vi "Identificação MIMO.vi"(6 "System Order":i32=4, 7 "Remove Trend":bool, 8 "Init Pump 2 voltage":dbl=3.0 min=0.0 format="%.2f", 9 "Init Pump 1 voltage":dbl=3.0 min=0.0 format="%.2f", 11 "Stimulus and Response Signal":dbl[][](array[numeric])) -> (0 "Acquired and identification signals":dbl[][](array[numeric]), 1 "output 2":dbl[][](graph) caption="Output H2", 2 "output 1":dbl[][](graph) caption="Output H1", 3 "Estimated MIMO State-space Model":picture, 5 "system model out":T1={"attributes"={"version"="1.0", "model type"=0, "input names"=[], "output names"=[], "notes"=""}, "coefficients"={"A "=[], "B"=[], "F"=[], "C"=[], "D"=[]}, "std deviations"={"A "=[], "B"=[], "F"=[], "C"=[], "D"=[]}, "coefficients covariance"=[], "noise variance"=[], "fs"=0.0, "system info"={"number of inputs"=0, "number of outputs"=0, "A order"=[], "B order"=[], "F order"=[], "C order"=[], "D order"=[], "Delays"=[]}, "kalman gain"=[], "initial state"=[], "trans func"=[], "zeros-poles"=[], "std of trans func"=[], "std of zeros-poles"=[], "trans func (noise)"=[], "std of trans func (noise)"=[], "zeros-poles (noise)"=[], "std of zeros-poles (noise)"=[], "Symbolic State Space Model"={"Symbolic A"=[], "Symbolic B"=[], "Symbolic C"=[], "Symbolic D"=[], "Symbolic K"=[], "Symbolic Initial State"=[]}, "delay"=[], "variables"=[], "grey trans func spec"={"orders of TF model"={" num order"=1, "den order"=2}, "# of zeros/poles at origin"={"zeros/poles"=1, "number "=0}, "delay initial?"=FALSE, "gain initial?"=FALSE}} {"grey trans func spec"."# of zeros/poles at origin"."zeros/poles" items=["zeros", "poles"]; "std of zeros-poles (noise)"."gain" format="%.2f"; "std of zeros-poles (noise)"."poles" format="%.2f"; "std of zeros-poles (noise)"."zeros" format="%.2f"; "zeros-poles (noise)"."gain" format="%.2f"; "zeros-poles (noise)"."poles" format="%.2f"; "zeros-poles (noise)"."zeros" format="%.2f"; "std of trans func (noise)"."alphas" format="%.2f"; "std of trans func (noise)"."betas" format="%.2f"; "trans func (noise)"."alphas" format="%.2f"; "trans func (noise)"."betas" format="%.2f"; "std of zeros-poles"."gain" format="%.2f"; "std of zeros-poles"."poles" format="%.2f"; "std of zeros-poles"."zeros" format="%.2f"; "std of trans func"."alphas" format="%.2f"; "std of trans func"."betas" format="%.2f"; "zeros-poles"."gain" format="%.2f"; "zeros-poles"."poles" format="%.2f"; "zeros-poles"."zeros" format="%.2f"; "trans func"."alphas" format="%.2f"; "trans func"."betas" format="%.2f"; "fs" format="%.2f"; "std deviations"."A" format="%.2f"; "std deviations"."D" format="%.2f"; "std deviations"."C" format="%.2f"; "std deviations"."F" format="%.2f"; "std deviations"."B" format="%.2f"; "coefficients"."A" format="%.2f"; "coefficients"."D" format="%.2f"; "coefficients"."C" format="%.2f"; "coefficients"."F" format="%.2f"; "coefficients"."B" format="%.2f"; "attributes"."model type" items=["Undefined", "AR", "ARX (SISO)", "ARX (MISO)", "ARX (MIMO)", "ARMAX (SISO)", "ARMAX (MISO)", "Output-Error (SISO)", "Output-Error (MISO)", "Box-Jenkins (SISO)", "Box-Jenkins (MISO)", "General Linear (SISO)", "General Linear (MISO)", "State-Space (SISO)", "State-Space (MISO)", "State-Space (MIMO)", "Transfer Function (SISO)", "Transfer Function (MISO)", "Transfer Function (MIMO)", "Zero-Pole-Gain (SISO)", "Zero-Pole-Gain (MISO)", "Zero-Pole-Gain (MIMO)"]})   [LabVIEW 2017]
uses:
  <vilib>/addons/System Identification/Model Typedefs.llb/si_generic model.ctl
  <vilib>/addons/System Identification/Model Typedefs.llb/SI Model Type.ctl
  <vilib>/addons/System Identification/Model Typedefs.llb/si_variables.ctl
  <vilib>/addons/System Identification/Data Preprocess.llb/SI Split Signal (MIMO Array).vi
  <vilib>/addons/System Identification/Data Preprocess.llb/SI Remove Trend (MIMO Array).vi
  <vilib>/addons/System Identification/Parametric Estimation.llb/SI Estimate State-space Model (MIMO Array).vi
  <vilib>/addons/System Identification/Model Analysis.llb/SI Model Simulation (MIMO Array).vi
  <vilib>/addons/System Identification/NI_SysID.lvlib
panel:
  out "responses":dbl[][](array[numeric])
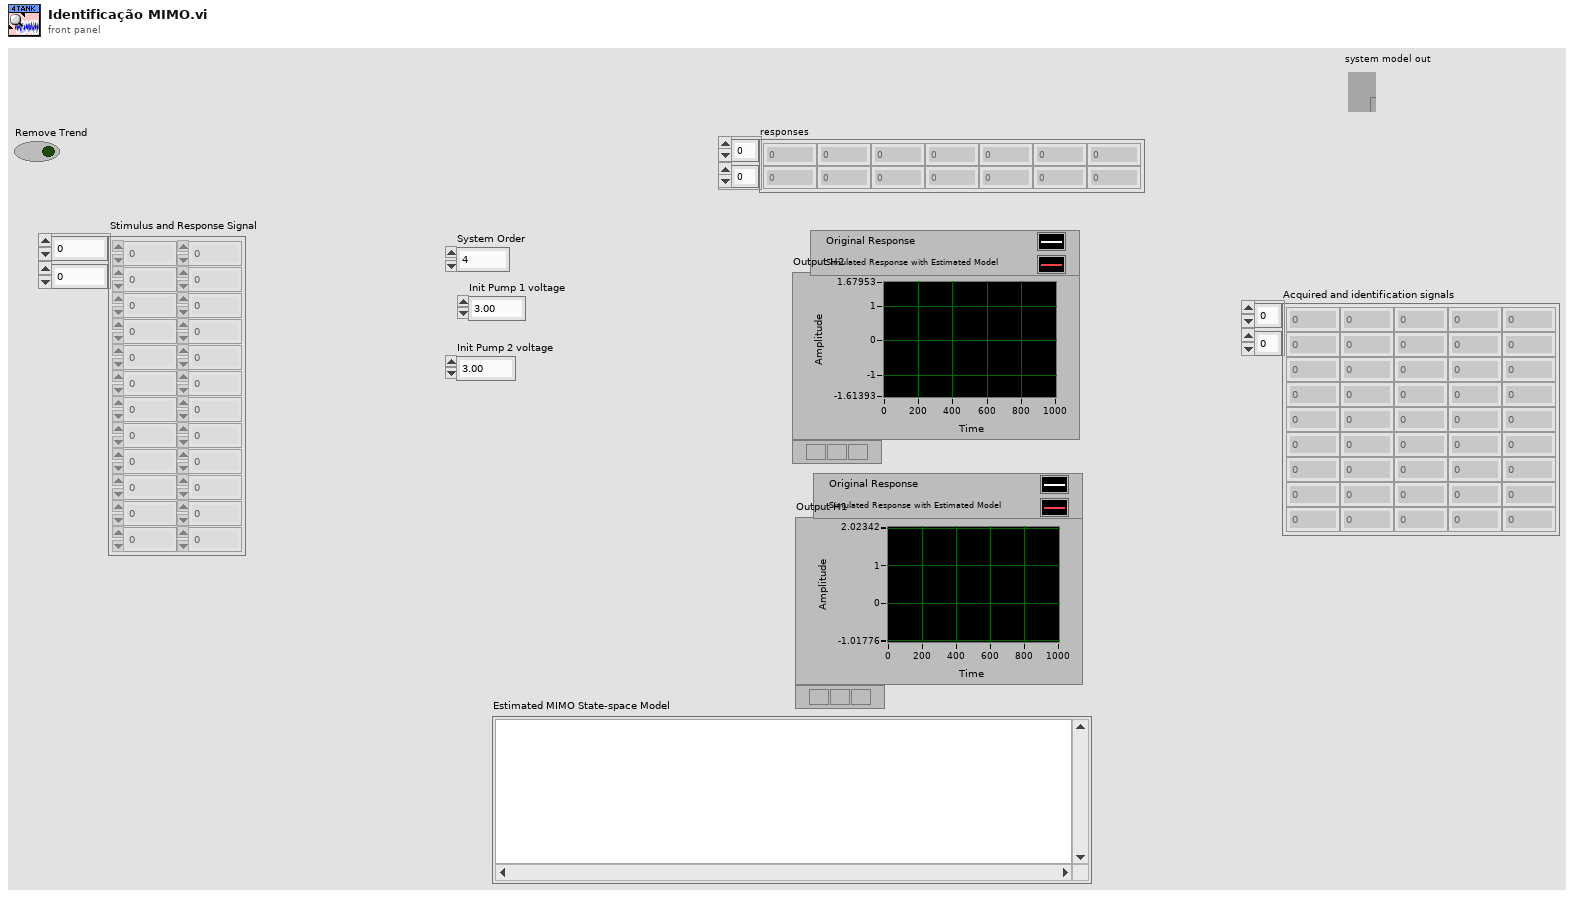
[diagram p1: front panel]
types:
  T1 = typedef "NI_SysID.lvlib/si_generic model.ctl" = cluster{"attributes":cluster{"version":string, "model type":T2, "input names":string[], "output names":string[], "notes":string}, "coefficients":cluster{"A ":dbl[][][], "B":dbl[][][], "F":dbl[][][], "C":dbl[][][], "D":dbl[][][]}, "std deviations":cluster{"A ":dbl[][][], "B":dbl[][][], "F":dbl[][][], "C":dbl[][][], "D":dbl[][][]}, "coefficients covariance":dbl[][][], "noise variance":dbl[][], "fs":dbl, "system info":cluster{"number of inputs":i32, "number of outputs":i32, "A order":i32[][], "B order":i32[][], "F order":i32[][], "C order":i32[][], "D order":i32[][], "Delays":i32[][]}, "kalman gain":dbl[][], "initial state":dbl[], "trans func":cluster{"betas":dbl[], "alphas":dbl[]}[][], "zeros-poles":cluster{"zeros":cdb[], "poles":cdb[], "gain":dbl}[][], "std of trans func":cluster{"betas":dbl[], "alphas":dbl[]}[][], "std of zeros-poles":cluster{"zeros":cdb[], "poles":cdb[], "gain":dbl}[][], "trans func (noise)":cluster{"betas":dbl[], "alphas":dbl[]}[][], "std of trans func (noise)":cluster{"betas":dbl[], "alphas":dbl[]}[][], "zeros-poles (noise)":cluster{"zeros":cdb[], "poles":cdb[], "gain":dbl}[][], "std of zeros-poles (noise)":cluster{"zeros":cdb[], "poles":cdb[], "gain":dbl}[][], "Symbolic State Space Model":cluster{"Symbolic A":string[][], "Symbolic B":string[][], "Symbolic C":string[][], "Symbolic D":string[][], "Symbolic K":string[][], "Symbolic Initial State":string[]}, "delay":dbl[][], "variables":T3, "grey trans func spec":cluster{"orders of TF model":cluster{" num order":i32, "den order":i32}, "# of zeros/poles at origin":cluster{"zeros/poles":u16, "number ":i32}, "delay initial?":bool, "gain initial?":bool}}
  T2 = typedef "NI_SysID.lvlib/SI Model Type.ctl" = u16
  T3 = typedef "NI_SysID.lvlib/si_variables.ctl" = cluster{"name":string, "initial guess":dbl, "upper limit":dbl, "lower limit":dbl, "value":dbl}[]
  T4 = cluster{"D matrix?":bool, "K matrix?":bool, "initial states?":bool}
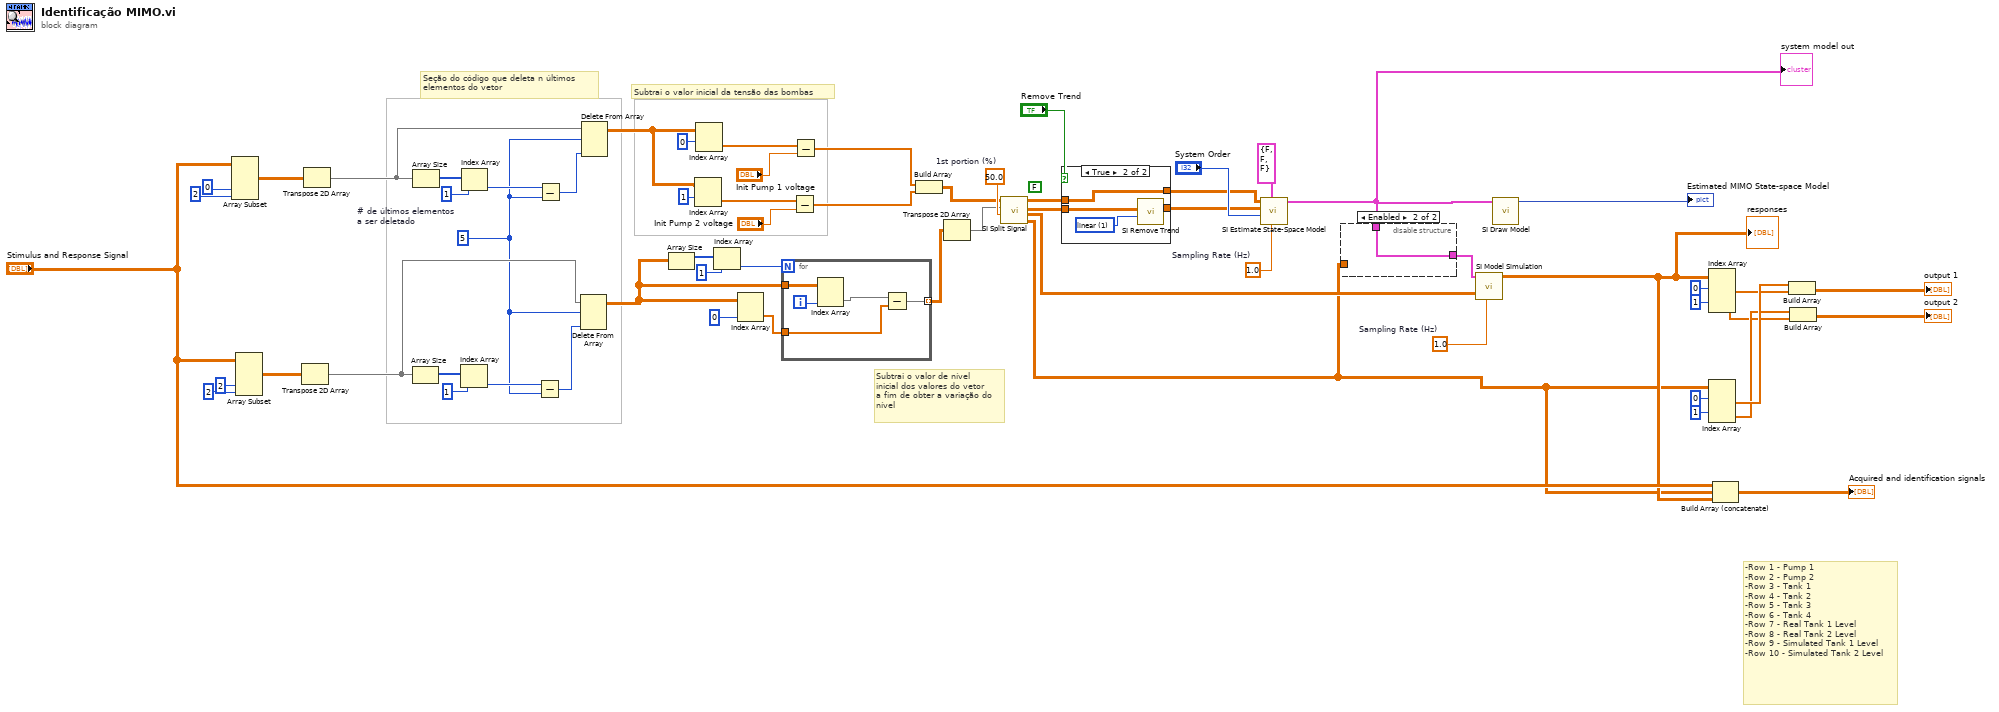
[diagram p0: block diagram]
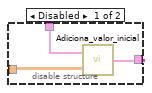
[diagram p3: hidden frame]
diagram:
  w9 = 1.0  # Sampling Rate (Hz)
  (unwired) FALSE
  w12 = 1.0  # Sampling Rate (Hz)
  w22 = 5  # # de últimos elementos  a ser deletado
  w55 = 50.0  # 1st portion (%)
  # "-Row 1 - Pump 1\n-Row 2 - Pump 2\n-Row 3 - Tank 1\n-Row 4 - Tank 2\n-Row 5 - Tank 3\n-Row 6 - Tank 4\n-Row 7 - Real Tank 1 Level\n-Row 8 - Real Tank 2 Level\n-Row 9 - Simulated Tank 1 Level\n-Row 10 - Simulated Tank 2 Level"
  # "Subtrai o valor inicial da tensão das bombas"
  # "Seção do código que deleta n últimos \nelementos do vetor"
  # "Subtrai o valor de nível \ninicial dos valores do vetor\na fim de obter a variação do\nnível"
  n1 = Array Subset(array="Stimulus and Response Signal", index (col)=0 ("index"), length (col)=2 ("length")) -> (w17:dbl[][])  [unwired: 2 in]
  n2 = Array Subset(array="Stimulus and Response Signal", index (col)=2 ("index"), length (col)=2 ("length")) -> (w16:dbl[][])  [unwired: 2 in]
  n3 = Transpose 2D Array(2D array=w16) -> (transposed array=w37:dbl[][])
  n4 = Transpose 2D Array(2D array=w17) -> (transposed array=w38:dbl[][])
  n5 = Array Size(array=w37) -> (size(s)=w53:i32[])
  n6 = Array Size(array=w38) -> (size(s)=w50:i32[])
  n7 = Index Array(array=w53, index=1) -> (element=w52:i32)
  n8 = Index Array(array=w50, index=1) -> (element=w51:i32)
  n9 = Subtract(x=w52, y=w22) -> (x-y=w34:i32)
  n10 = Subtract(x=w51, y=w22) -> (x-y=w33:i32)
  n11 = Delete From Array(array=w37, length=w22, index (col)=w34) -> (array with subset deleted=w28:dbl[][])  [unwired: 1 in, 1 out]
  n12 = Delete From Array(array=w38, length=w22, index (col)=w33) -> (array with subset deleted=w40:dbl[][])  [unwired: 1 in, 1 out]
  n13 = Array Size(array=w28) -> (size(s)=w27:i32[])
  n14 = Index Array(array=w40, index (row)=1 ("index")) -> (element=w48:dbl[])  [unwired: 1 in]
  n15 = Index Array(array=w40, index (row)=0 ("disabled index (col)")) -> (element=w49:dbl[])  [unwired: 1 in]
  n16 = Index Array(array=w27, index=1) -> (element=w25:i32)
  n17 = Index Array(array=w28, index (col)=0 ("index (row)")) -> (element=w54:dbl[])  [unwired: 1 in]
  n18 = for {
    N: w25 -> [_]
    tunnel: w54 -> [w68]
    tunnel: w28 -> [w66]
    tunnel: [w67] -> w23 mode=indexing
    i -> [w65]
    n19 = Index Array(array=w66, index (col)=w65) -> (element=w64:dbl[])  [unwired: 1 in]
    n20 = Subtract(x=w64, y=w68) -> (x-y=w67:dbl[])
  }
  n21 = Subtract(x=w48, y="Init Pump 2 voltage") -> (x-y=w47:dbl[])
  n22 = Subtract(x=w49, y="Init Pump 1 voltage") -> (x-y=w39:dbl[])
  n23 = Build Array(w39, w47) -> (w30:dbl[][])
  n24 = Transpose 2D Array(2D array=w23) -> (transposed array=w24:dbl[][])
  n25 = call-poly <vilib>:"SI Split Signal.vi"("1st portion (%)"=w55, "response signals in"=w24, "stimulus signals in"=w30) -> ("response signals 2"=w1:dbl[][], "stimulus signals 2"=w56:dbl[][], "response signals 1"=w7:dbl[][], "stimulus signals 1"=w8:dbl[][])  [unwired: 5 in]
  n26 = case shown="True" "Remove Trend" {
    tunnel: w8 -> [w69 w71]
    tunnel: w7 -> [w70 w74]
    tunnel: [w70 w73] -> w6
    tunnel: [w69 w71] -> w4
    frame False {
    }
    frame True {
      w72 = 1 items=["mean", "linear"] ("trend type")
      n27 = call-poly <vilib>:"SI Remove Trend.vi"("trend type"=w72, "response signals in"=w74) -> ("response signals out"=w73:dbl[][])  [unwired: 5 in, 4 out]
    }
  }
  n28 = call-poly <vilib>:"SI Estimate State-Space Model.vi"("sampling rate (Hz)"=w9, "structure selector"=T4 {"D matrix?"=FALSE, "K matrix?"=FALSE, "initial states?"=FALSE}, "number of states"="System Order", "response signals"=w6, "stimulus signals"=w4) -> ("system model out"=w3:T1)  [unwired: 1 in, 5 out]
  "system model out" <- w3
  n29 = disable-structure shown="Enabled" {
    disable-tunnel: w1 -> [w76 _]
    disable-tunnel: [w75 w78] -> w2
    disable-tunnel: w3 -> [w77 w78]
    frame Disabled {
      n30 = call "Adiciona_valor_inicial.vi"("Array"=w76, "system model in"=w77) -> ("system model out"=w75:T1)
    }
    frame Enabled {
    }
  }
  n31 = call-poly <vilib>:"SI Model Simulation.vi"("sampling rate (Hz)"=w12, "stimulus signals"=w56, "system model"=w2) -> ("responses"=w14:dbl[][])  [unwired: 6 in, 2 out]
  "responses" <- w14
  n32 = call <vilib>:"SI Draw Model.vi"("system model"=w3) -> ("model"=→"Estimated MIMO State-space Model":picture)  [unwired: 8 in, 2 out]
  n33 = Index Array(array=w14, index (row) #1=0 ("disabled index (col)"), index (row) #2=1 ("index (col)")) -> (element #1=w42:dbl[], element #2=w41:dbl[])  [unwired: 2 in]
  n34 = Index Array(array=w1, index (row) #1=0 ("disabled index (col)"), index (row) #2=1 ("index (col)")) -> (element #1=w44:dbl[], element #2=w43:dbl[])  [unwired: 2 in]
  n35 = Build Array (concatenate)("Stimulus and Response Signal", w1, w14) -> (→"Acquired and identification signals":dbl[][])
  n36 = Build Array(w44, w42) -> (→"output 1":dbl[][])
  n37 = Build Array(w43, w41) -> (→"output 2":dbl[][])
